vi "SLSC Command Loop Timer.vi"(11 "inputs.Sample Rate (S/s)":u32=10000) -> (1 "Actual Loop Ticks":u32, 2 "oclk freq":u32, 3 "oclk div":u32)   [LabVIEW 2014, in "SLSC FPGA Toolkit.lvlib"]
uses:
  SLSC FPGA Toolkit.lvlib
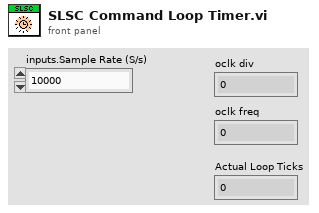
[diagram p1: front panel]
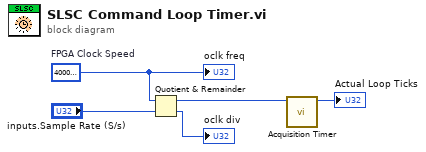
[diagram p0: block diagram]
diagram:
  w4 = u32 40000000  # FPGA Clock Speed
  n1 = Quotient & Remainder(x=w4, y="inputs.Sample Rate (S/s)") -> (x-y*floor(x/y)=w1:u32, floor(x/y)=→"oclk div":u32)
  n2 = call <vilib>:"Acquisition Timer.vi"("Loop Time (Ticks)"=w1) -> ("Actual Time (Ticks)"=→"Actual Loop Ticks":u32)  [unwired: 10 in]
  "oclk freq" <- w4
